vi "3A PWM MotorControl.vi"() -> ()   [LabVIEW 2011]
uses:
  <vilib>/rvi/interface/nirviOpenFPGA/nirviOpenFPGA.xnode
  <vilib>/rvi/interface/nirviCloseFPGA/nirviCloseFPGA.xnode
  FPGA/3A PWM MotorControl FPGA.vi
  <vilib>/rvi/interface/nirviReadWriteControl/nirviReadWriteControl.xnode
  2-Think/2 Globals/2 Global.vi
  FPGA Bitfiles/SailBot_FPGATarget_3APWMMotorContro_81FD9E83.lvbitx
  <vilib>/FPGAPlugInAG/cRIO-9113/niLvFpga_Open_cRIO-9113.vi
  <vilib>/rvi/errors/niLvFpgaMergeErrorWithErrorCode.vi
  <vilib>/rvi/errors/niLvFpgaAdjustHostInterfaceError.vi
  <vilib>/FPGAPlugInAG/cRIO-9113/niLvFpga_Close_cRIO-9113.vi
  2-Think/2 Typedefs/rudder angle.ctl
  2-Think/2 Typedefs/sail setpt.ctl
panel:
  in  "Rudder Range":dbl=50.0
  in  "Rudder Trim":dbl(slide) scale=-20.0..20.0
  out "Sail Position":T1
  out "Rudder Angle":T2
  in  "stop":bool
  out "error out":errorcluster
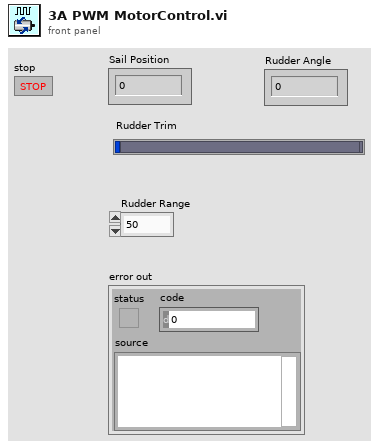
[diagram p1: front panel]
types:
  T1 = typedef "sail setpt.ctl" = dbl
  T2 = typedef "rudder angle.ctl" = dbl
  T3 = typedef "setpoints to boat.ctl" = cluster{"Sail Position":T1, "Rudder Angle":T2}
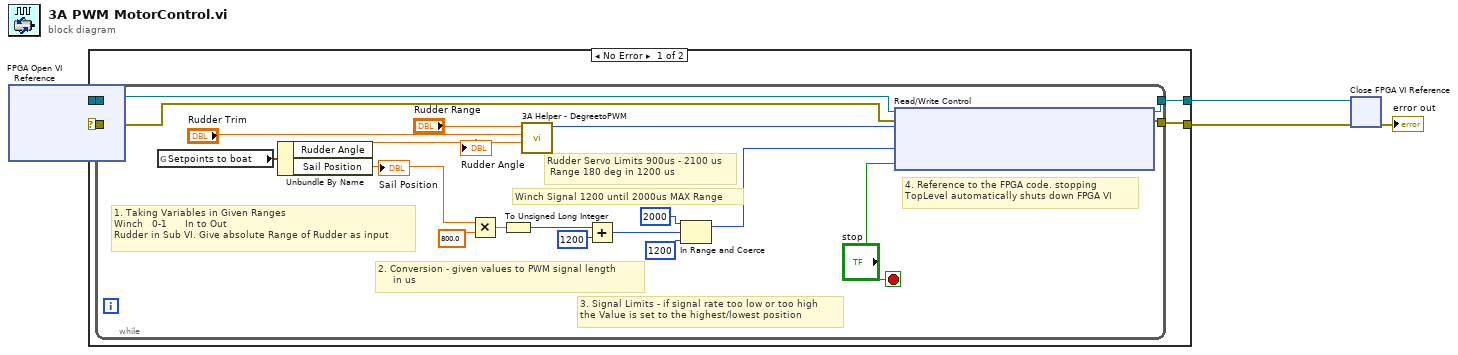
[diagram p0: block diagram]
diagram:
  n1 = xnode "FPGA Open VI Reference"() -> ("FPGA VI Reference Out"=w4:refnum<k20>, "error out"=w3:errorcluster)  [unwired: 2 in]
  n2 = case shown="No Error" w3 {
    selector: w3 -> [w9 w29]
    tunnel: [w6 w30] -> w2
    tunnel: [w7 w29] -> w1
    tunnel: w4 -> [w8 w30]
    frame No Error {
      n3 = while {
        tunnel: w8 -> [w24]
        tunnel: w9 -> [w25]
        tunnel: [w23] -> w7
        tunnel: [w22] -> w6
        stop <- "stop" stop-if-true
        # "Rudder Servo Limits 900us - 2100 us\n Range 180 deg in 1200 us"
        # "1. Taking Variables in Given Ranges\nWinch   0-1      In to Out\nRudder in Sub VI. Give absolute Range of Rudder as input"
        # "2. Conversion - given values to PWM signal length\n     in us"
        # "3. Signal Limits - if signal rate too low or too high \nthe Value is set to the highest/lowest position"
        # "4. Reference to the FPGA code. stopping \nTopLevel automatically shuts down FPGA VI"
        # "Winch Signal 1200 until 2000us MAX Range"
        n4 = global read "2 Global.vi" "Setpoints to boat"() -> (w14:T3)
        n5 = Unbundle By Name(w14) -> ("Rudder Angle"=w13:T2, "Sail Position"=w11:T1)
        "Rudder Angle" <- w13
        "Sail Position" <- w11
        n6 = Multiply(x=w11, y=800.0) -> (x*y=w28:T1)
        n7 = To Unsigned Long Integer(number=w28) -> (unsigned 32bit integer=w27:u32)
        n8 = call "3A Helper - DegreetoPWM.vi"("Rudder Angle"=w13, "Rudder Trim"="Rudder Trim", "Rudder Range (deg)"="Rudder Range") -> ("Servo Position (us)"=w19:u32)  [unwired: 8 in]
        n9 = Add(x=w27, y=u32 1200) -> (x+y=w18:u32)
        n10 = In Range and Coerce(upper limit=u32 2000, x=w18, lower limit=u32 1200) -> (coerced(x)=w15:u32)  [unwired: 1 out]
        n11 = xnode "Read/Write Control"("FPGA VI Reference In"=w24, "error in"=w25, "SERVO 2 Duty in Ticks"=w19, "SERVO 1 Duty in Ticks"=w15, "stop PWM"="stop") -> ("FPGA VI Reference Out"=w22:refnum<k20>, "error out"=w23:errorcluster)
      }
    }
    frame Error {
      # "Error occurred. Do not run."
    }
  }
  n12 = xnode "Close FPGA VI Reference"("FPGA VI Reference In"=w2, "error in"=w1) -> ("error out"=→"error out":errorcluster)
